vi "Read_Camera.vi"(0 "error in":errorcluster, 2 "Camera":T2, 3 "node":string) -> (1 "error out":errorcluster, 4 "image out":T3 {"Dialogs" format="%.0b"})   [LabVIEW 2010]
doc: "Get an image from one of Baxter's hand cameras. \n\nIt is highly recommended that you are connected to baxter via ethernet rather than over wireless when doing this."
uses:
  ROS/Code/SubVIs/_ROSDirection.ctl
  ROS/Code/Console/Servers/ServerSubs/TopicDef.ctl
  ImageProcessing/QTLIB_2595_LV86/QT_Image.ctl
  ROS/Code/SubVIs/BaxterCamera.ctl
panel:
  out "ROS Image":T1
  out "image":picture
  out "Reply":string
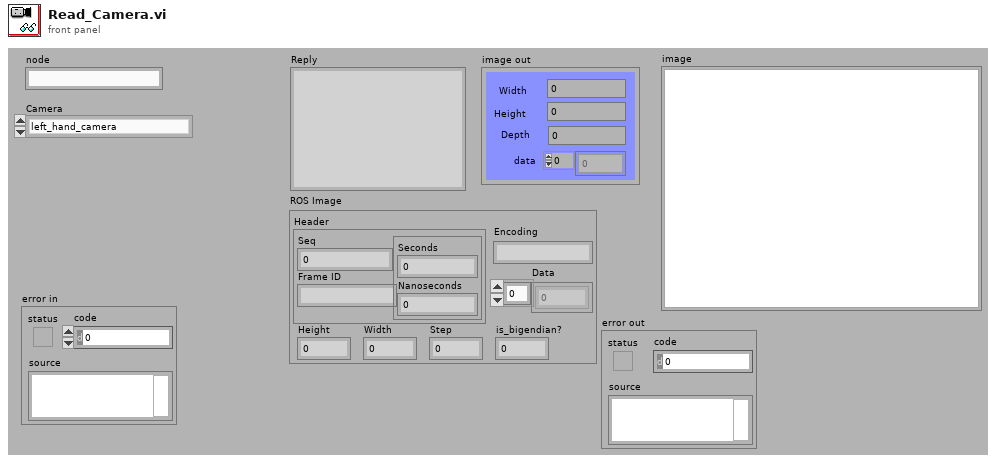
[diagram p1: front panel]
types:
  T1 = cluster{"Header":cluster{"Seq":u32, "Frame ID":string, cluster{"Seconds":i32, "Nanoseconds":i32}}, "Height":u32, "Width":u32, "is_bigendian?":u8, "Step":u32, "Data":u8[], "Encoding":string}
  T2 = typedef "BaxterCamera.ctl" = enum16{"left_hand_camera", "right_hand_camera", "head_camera"}
  T3 = typedef "QT_Image.ctl" = cluster{"Width":i32, "Height":i32, "Depth":i32, "data":u8[], "Compressed data":u8[], "Color table":u32[], "Duration":i32, "Options":i32, "Timestamp":i32, "ID":i32, "Reserved":i32, "Dialogs":u32}
  T4 = typedef "TopicDef.ctl" = cluster{"Topic":string, "Type":string, "Action":T5, "Update (ms)":u16, "write queue":u16}
  T5 = typedef "_ROSDirection.ctl" = enum16{"Node", "Publisher", "Subscriber", "Service Client"}
  T6 = typedef "_ROSControl.ctl" = cluster{"topic port":u16, "Node":string, "topic":string, "type":string, "node port":u32, "error ":errorcluster, "Direction":T5, "APIs":string[], "Update (ms)":u16, "write queue":u16}
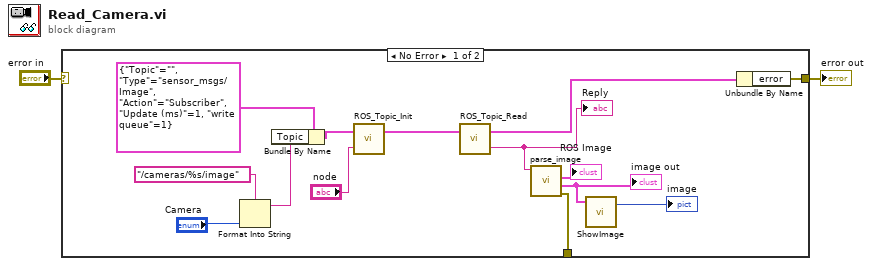
[diagram p0: block diagram]
diagram:
  n1 = case shown="No Error" "error in" {
    selector: "error in" -> [_ w17]
    tunnel: [w16 w17] -> w2
    tunnel: [w9 _] -> _
    frame No Error {
      n2 = Format Into String(format string="/cameras/%s/image" ("topic"), "Camera") -> (resulting string=w4:string)  [unwired: 2 in, 1 out]
      n3 = Bundle By Name(cluster=T4 {"Topic"="", "Type"="sensor_msgs/Image", "Action"=enum."Subscriber", "Update (ms)"=1, "write queue"=1} ("Definitions"), "Topic"=w4) -> (w3:T4)
      n4 = call "ROS_Topic_Init.vi"("node"="node", "Definitions"=w3) -> ("ROS out"=w14:T6)  [unwired: 1 in]
      n5 = call "ROS_Topic_Read.vi"("ROS in"=w14) -> ("Reply"=w11:string, "ROS out"=w13:T6)  [unwired: 1 in]
      "Reply" <- w11
      n6 = call "parse_image.vi"("msg in"=w11) -> ("error out"=w9:errorcluster, "Image Out"=w8:T3, "ROS Image"=→"ROS Image":T1)  [unwired: 3 in, 1 out]
      "image out" <- w8
      n7 = call "ShowImage.vi"("Image"=w8) -> ("image"=→"image":picture)  [unwired: 2 in, 1 out]
      n8 = Unbundle By Name(w13) -> ("error"=w16:errorcluster)
    }
    frame Error {
    }
  }
  "error out" <- w2
